vi "Ke24xx Enable_Disable Source Output.vi"(3 "error in (no error)":errorcluster, 4 "state":bool, 5 "instrument handle":refnum<visa-resource-name>) -> (0 "error out":errorcluster, 1 "status":i32 format="%.0x", 2 "instrument handle out":refnum<visa-resource-name>)   [LabVIEW 2009]
doc: "This function is used to enable or disable the source output. See instruments user's manual (2400S-900-01 Rev. D) page 18-51 for more details on this operation.\n\nDefinition :\n\nViStatus CVIFUNC Ke24xx_EnableSource (\n ViSession instrumentHandle,\n ViBoolean state);\n\n\nParameter :\n\ninstrumentHandle : ViSession value returned from the Initialize function.\n\nstate : Set this parameter to ViTrue or ViFalse to enable or disable the source output."
uses:
  <instrlib>/Ke24xx/ke24xx.dll
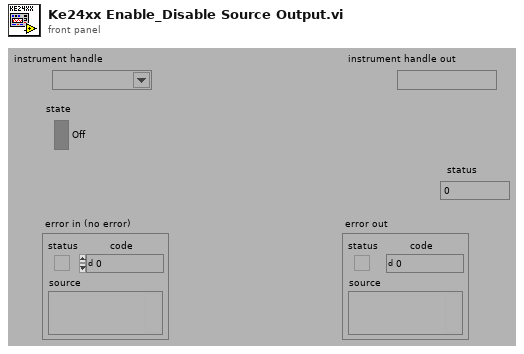
[diagram p1: front panel]
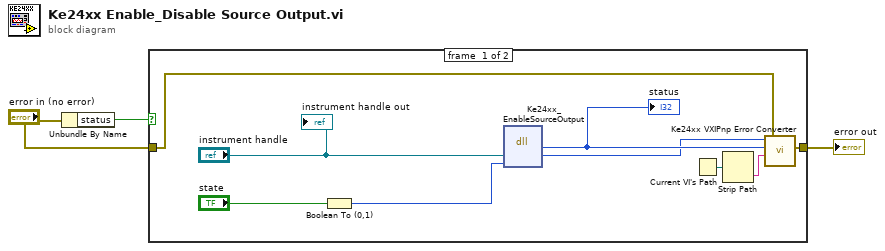
[diagram p0: block diagram]
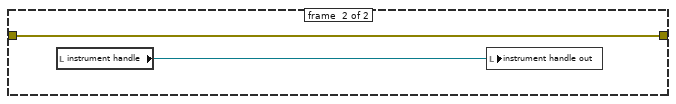
[diagram p2: hidden frame]
diagram:
  n1 = Unbundle By Name("error in (no error)") -> ("status"=w2:bool)
  n2 = case shown="False" w2 {
    tunnel: "error in (no error)" -> [w6 w14]
    tunnel: [w7 w14] -> w1
    frame #0 {
      n3 = Boolean To (0,1)(Boolean="state") -> (0, 1=w9:i16)
      n4 = dll-call lib="C:/Program Files/National Instruments/LabVIEW 2009/instr.lib/Ke24xx/ke24xx.dll" fn="Ke24xx_EnableSourceOutput"("instrument handle"="instrument handle", "state"=w9) -> ("status"=w10:i32, "instrument handle"=w8:u32)  [unwired: 4 in, 2 out]
      "status" <- w10
      n5 = Current VI's Path() -> (path=w5:path)
      n6 = Strip Path(path=w5) -> (name=w4:string)  [unwired: 1 out]
      n7 = call <instrlib>:"Ke24xx VXIPnp Error Converter.vi"("error in (no error)"=w6, "name of VI (\"\")"=w4, "CVI error code (0)"=w10, "instrument handle"=w8) -> ("error out"=w7:errorcluster)  [unwired: 1 out]
      "instrument handle out" <- "instrument handle"
    }
    frame #1 {
      n8 = local read "instrument handle"() -> (w13:refnum<visa-resource-name>)
      n9 = local write "instrument handle out"(w13) -> ()
    }
  }
  "error out" <- w1
